vi "Load Theme.vi"(8 "error in":errorcluster, 11 "File Path":path) -> (0 "error out":errorcluster, 3 "Theme":refnum<class "Theme.lvclass">)   [LabVIEW 2021, in "Theme.lvclass"]
doc: "Load a theme from file\n\n<b>Code Developed By:</b> +\nDaniel Coons +\nhttps://github.com/danielcoons/tsc-pop-up"
uses:
  Theme.lvclass
  Popup/PopUp Theme Global.vi
  Theme.lvclass/Theme.ctl
  Popup/Popup.lvclass
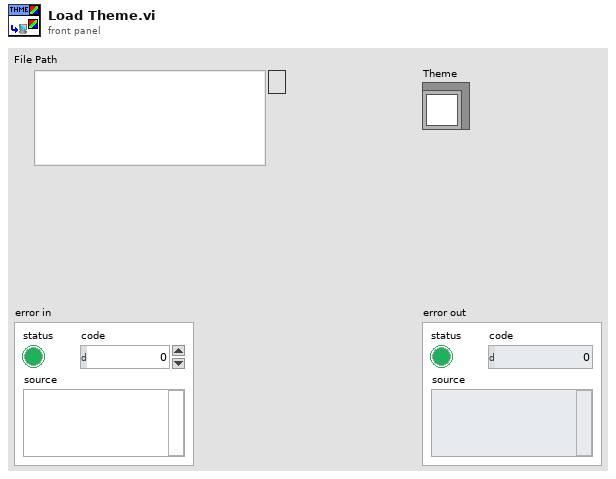
[diagram p1: front panel]
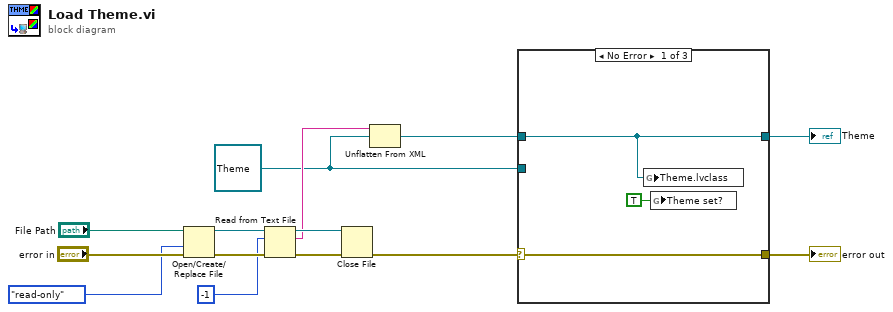
[diagram p0: block diagram]
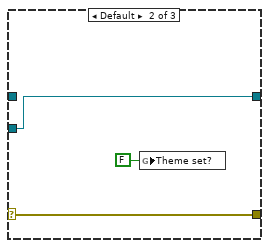
[diagram p2: hidden frame]
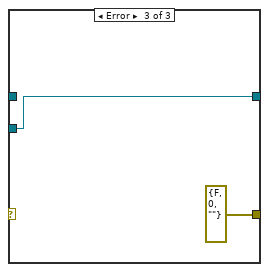
[diagram p3: hidden frame]
diagram:
  w2 = refnum<class "Theme.lvclass"> refnum ("Theme")
  n1 = Open/Create/Replace File(file path (use dialog)="File Path", error in="error in", access (0:read/write)=enum16{"read/write", "read-only", "write-only"}."read-only") -> (refnum out=w9:refnum<file>, error out=w13:errorcluster)  [unwired: 3 in, 1 out]
  n2 = Read from Text File(file (use dialog)=w9, count=-1, error in=w13) -> (refnum out=w8:refnum<file>, text=w6:string, error out=w12:errorcluster)  [unwired: 1 in, 1 out]
  n3 = Close File(refnum=w8, error in=w12) -> (error out=w5:errorcluster)  [unwired: 1 out]
  n4 = Unflatten From XML(xml string=w6, type=w2) -> (value=w3:refnum<class "Theme.lvclass">)  [unwired: 1 in, 1 out]
  n5 = case shown="No Error" w5 {
    selector: w5 -> [w17 w20 _]
    tunnel: [w17 w20 errorcluster {"status"=FALSE, "code"=0, "source"=""} ("error IO")] -> w4
    tunnel: w3 -> [w16 _ _]
    tunnel: [w16 w19 w21] -> w1
    tunnel: w2 -> [_ w19 w21]
    frame No Error {
      n6 = global write "PopUp Theme Global.vi" "Theme.lvclass"(w16) -> ()
      n7 = global write "PopUp Theme Global.vi" "Theme set?"(TRUE ("Theme set?")) -> ()
    }
    frame Default {
      n8 = global write "PopUp Theme Global.vi" "Theme set?"(FALSE ("Theme set?")) -> ()
    }
    frame Error {
    }
  }
  "error out" <- w4
  "Theme" <- w1
